vi "WPI_I2CClose.vi"(8 "error in (no error)":errorcluster, 11 "I2CDevRef":T1={"DevStatus"={"status"=FALSE, "code"=0, "source"=""}, "Device Address"=0, "Handle"=0, "I2C Bus"=enum."Invalid"} {"Device Address" format="%.0x"}) -> (0 "error out":errorcluster)   [LabVIEW 2017]
doc: "Closes a reference to the I2C sensor you specify. Use this VI to close each I2C sensor reference that you open with the Open VI.\n\nThis software is licensed. Open the labview\\readme\\WPI Robotics Library Open Source License.txt file for more information."
uses:
  <vilib>/Rock Robotics/WPI/I2C/WPI_I2CDevRef.ctl
  <vilib>/Rock Robotics/SystemInterfaces/i2clib/i2c_bus.ctl
  <vilib>/Rock Robotics/WPI/SPI/WPI_SPIBusCacheOp.ctl
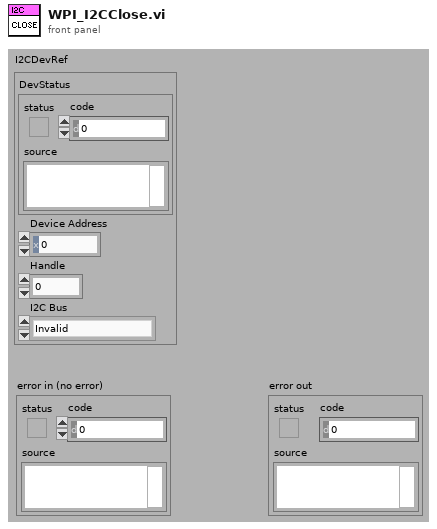
[diagram p1: front panel]
types:
  T1 = typedef "WPI_I2CDevRef.ctl" = cluster{"DevStatus":errorcluster, "Device Address":u8, "Handle":i32, "I2C Bus":T2}
  T2 = typedef "i2c_bus.ctl" = enum16{"I2C On-Board", "I2C MXP", "Invalid"}
  T3 = typedef "WPI_SPIBusCacheOp.ctl" = enum16{"Acquire", "Release", "Status"}
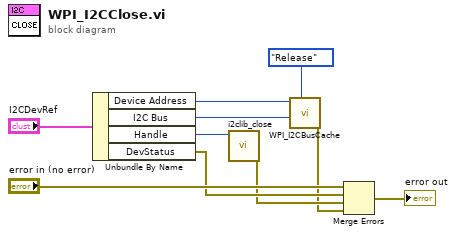
[diagram p0: block diagram]
diagram:
  n1 = Unbundle By Name("I2CDevRef") -> ("Device Address"=w2:u8, "I2C Bus"=w1:T2, "Handle"=w9:i32, "DevStatus"=w6:errorcluster)
  n2 = call <vilib>:"i2clib_close.vi"("I2C Reference"=w9) -> ("error out"=w5:errorcluster)  [unwired: 10 in]
  n3 = call <vilib>:"WPI_I2CBusCache.vi"("Operation"=WPI_SPIBusCacheOp."Release", "I2C Bus"=w1, "Device Address"=w2) -> ("error out"=w3:errorcluster)  [unwired: 6 in, 2 out]
  n4 = Merge Errors("error in (no error)", w6, w5, w3) -> (→"error out":errorcluster)
